vi "nirvififoEmulationGetNumberOfElementsToRead.vi"(5 "Width":i32=1024, 7 "ErrorIn":bool, 8 "Name":string="simul", 9 "Local? (F)":bool, 14 "Size":i32=1024, 15 "ref in wired":bool, 16 "Type":variant, 17 "Update Size?":bool) -> (24 "Number of Elements to Read":i32)   [LabVIEW 2017]
uses:
  <instcachedir>/0/nirviFifoEmulationQueueMgr_E5CAEC123FF24DC58D834DCA3CDAA9B5.lvgen/nirviFifoEmulationQueueMgr_E5CAEC123FF24DC58D834DCA3CDAA9B5_000.vi
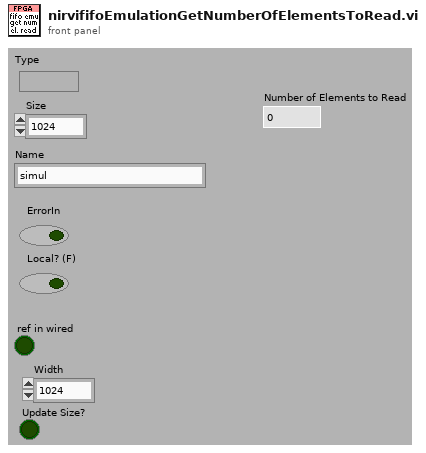
[diagram p1: front panel]
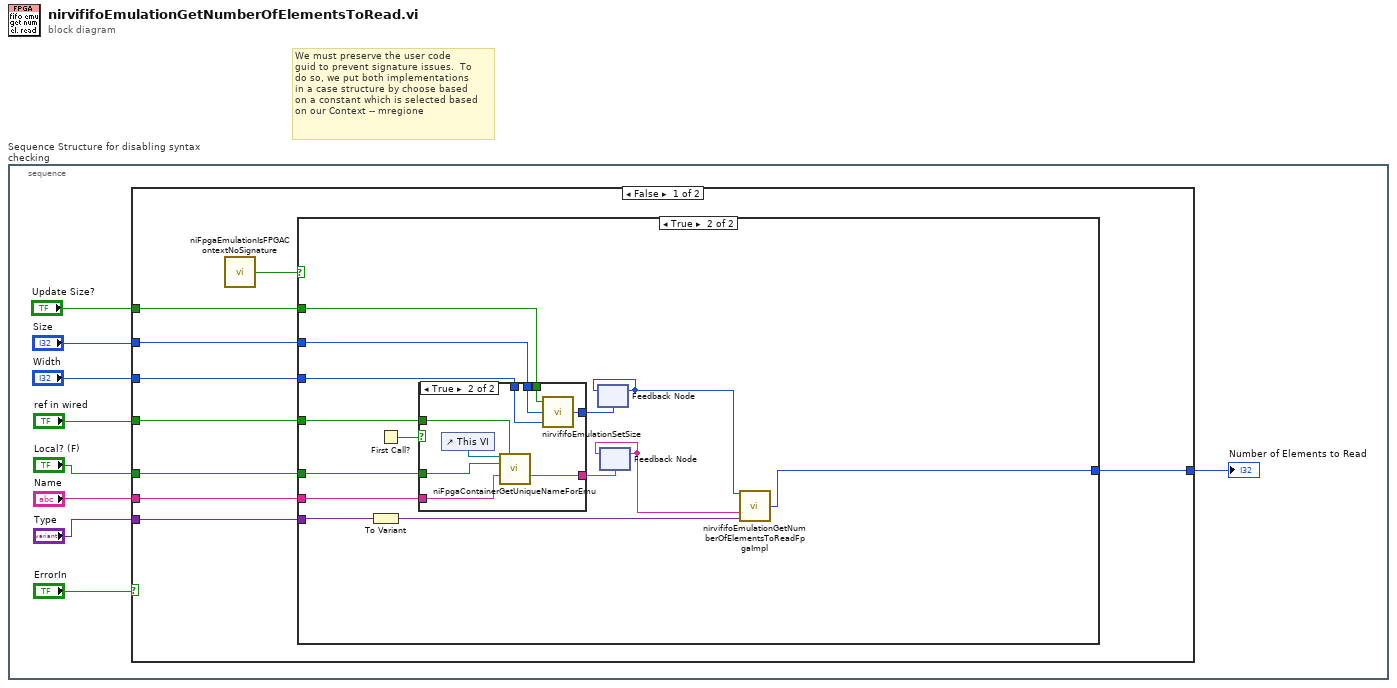
[diagram p0: block diagram]
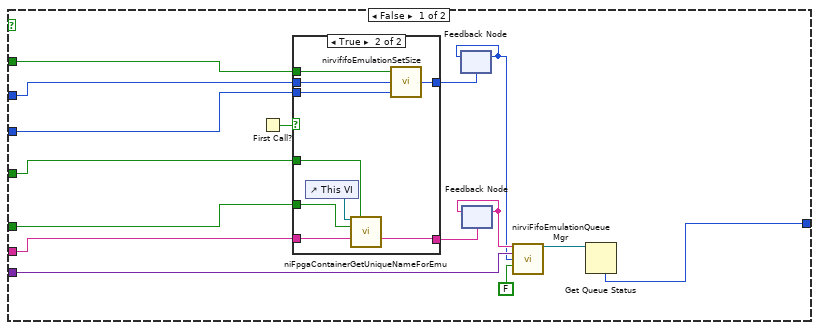
[diagram p2: hidden frame]
diagram:
  # "We must preserve the user code\nguid to prevent signature issues.  To\ndo so, we put both implementations\nin a case structure by choose based\non a constant which is selected based\non our Context -- mregione"
  n1 = stacked-sequence "Sequence Structure for disabling syntax checking" {
    frame #0 {
      n2 = case shown="False" "ErrorIn" {
        tunnel: "Name" -> [w17 _]
        tunnel: "ref in wired" -> [w15 _]
        tunnel: "Local? (F)" -> [w16 _]
        tunnel: "Size" -> [w14 _]
        tunnel: "Type" -> [w18 _]
        tunnel: [w13 _] -> w3
        tunnel: "Update Size?" -> [w12 _]
        tunnel: "Width" -> [w11 _]
        frame False {
          n3 = call <vilib>:"niFpgaEmulationIsFPGAContextNoSignature.vi"() -> ("Is Fpga Context?"=w10:bool)  [unwired: 15 in]
          n4 = case shown="True" w10 {
            tunnel: w18 -> [w22 w52]
            tunnel: w17 -> [w33 w48]
            tunnel: w16 -> [w32 w49]
            tunnel: w15 -> [w31 w50]
            tunnel: w14 -> [w30 w46]
            tunnel: [w29 w51] -> w13
            tunnel: w12 -> [w28 w47]
            tunnel: w11 -> [w27 w45]
            frame False {
              n5 = First Call?() -> (First Call?: T/F=w26:bool)
              n6 = case shown="True" w26 {
                tunnel: w33 -> [_ w39]
                tunnel: w30 -> [_ w42]
                tunnel: w32 -> [_ w38]
                tunnel: w31 -> [_ w36]
                tunnel: w27 -> [_ w41]
                tunnel: w28 -> [_ w40]
                tunnel: [_ w35] -> w25
                tunnel: [_ w34] -> w24
                frame False {
                }
                frame True {
                  n7 = control-ref of="This VI"() -> (w37:refnum<vi>)
                  n8 = call <vilib>:"niFpgaContainerGetUniqueNameForEmu.vi"("parent VI"=w37, "ref in wired"=w36, "local"=w38, "name in"=w39) -> ("name out"=w34:string)  [unwired: 11 in]
                  n9 = call <vilib>:"nirvififoEmulationSetSize.vi"("width"=w41, "Size"=w42, "Update?"=w40) -> ("Actual Size"=w35:i32)
                }
              }
              n10 = feedback #1(w25) -> (w21:i32)
              n11 = feedback-in #1(w21) -> ()
              n12 = feedback #2(w24) -> (w23:string)
              n13 = feedback-in #2(w23) -> ()
              n14 = call-generic <vilib>:"nirviFifoEmulationQueueMgr.vi"("FIFO Name"=w23, "Element"=w22, "Size"=w21, "Is Handshake?"=FALSE) -> ("FIFO"=w19:refnum<queue>)  [unwired: 11 in]
              n15 = Get Queue Status(queue=w19) -> (# elements in queue=w29:i32)  [unwired: 2 in, 7 out]
            }
            frame True {
              n16 = To Variant(anything=w52) -> (Variant=w53:variant)
              n17 = First Call?() -> (First Call?: T/F=w54:bool)
              n18 = case shown="True" w54 {
                tunnel: [_ w64] -> w55
                tunnel: w50 -> [_ w63]
                tunnel: w49 -> [_ w62]
                tunnel: w48 -> [_ w61]
                tunnel: w47 -> [_ w60]
                tunnel: w46 -> [_ w59]
                tunnel: [_ w58] -> w44
                tunnel: w45 -> [_ w57]
                frame False {
                }
                frame True {
                  n19 = control-ref of="This VI"() -> (w65:refnum<vi>)
                  n20 = call <vilib>:"niFpgaContainerGetUniqueNameForEmu.vi"("parent VI"=w65, "ref in wired"=w63, "local"=w62, "name in"=w61) -> ("name out"=w64:string)  [unwired: 11 in]
                  n21 = call <vilib>:"nirvififoEmulationSetSize.vi"("width"=w57, "Size"=w59, "Update?"=w60) -> ("Actual Size"=w58:i32)
                }
              }
              n22 = feedback #3(w44) -> (w43:i32)
              n23 = feedback-in #3(w43) -> ()
              n24 = feedback #4(w55) -> (w56:string)
              n25 = feedback-in #4(w56) -> ()
              n26 = call <vilib>:"nirvififoEmulationGetNumberOfElementsToReadFpgaImpl.vi"("Size"=w43, "Name"=w56, "Init Val"=w53) -> ("num to read"=w51:i64)  [unwired: 12 in]
            }
          }
        }
        frame True {
        }
      }
      "Number of Elements to Read" <- w3
    }
  }
